vi "Global_CMD to SM Data.vi"() -> ()   [LabVIEW 2017, in "Climber.lvlib"]
uses:
  Climber.lvlib
  Cluster_Cmd to SM Data.ctl
  ENUM_SM Cmd Select.ctl
panel:
  in  "Cmd Climb":T1
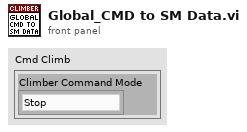
[diagram p1: front panel]
types:
  T1 = typedef "Climber.lvlib/Cluster_Cmd to SM Data.ctl" = cluster{"Climber Command Mode":T2}
  T2 = typedef "Climber.lvlib/ENUM_SM Cmd Select.ctl" = enum16{"Stop", "Auto Climb", "Manual", "No Command"}
diagram:
